vi "Serial_write_Read.vi"(8 "Error In":errorcluster caption="에러 입력", 10 "Command":string, 11 "VISA 리소스 이름":refnum<visa-resource-name>) -> (0 "Error Out":errorcluster caption="에러 출력", 2 "Response":T1, 3 "VISA 리소스 이름 출력":refnum<visa-resource-name>, 5 "bytes read":u32)   [LabVIEW 2015]
uses:
  MFC_Address.ctl
panel:
  out "연결된 문자열":string
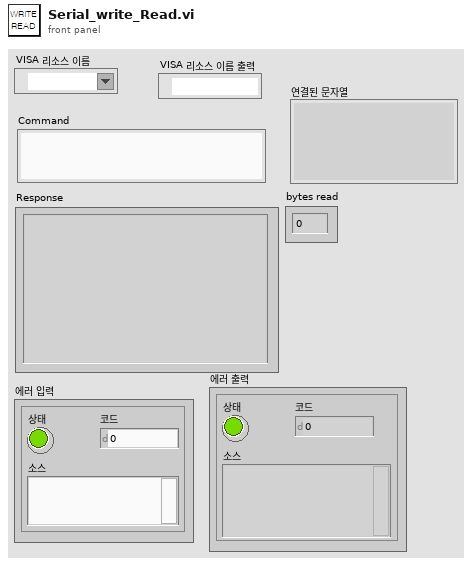
[diagram p1: front panel]
types:
  T1 = typedef "MFC_Address.ctl" = string
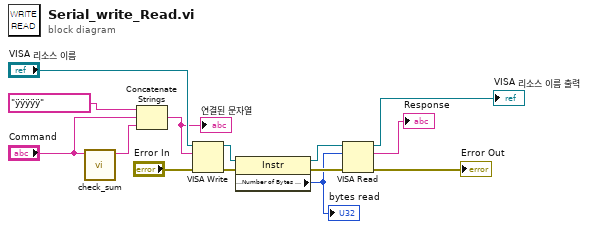
[diagram p0: block diagram]
diagram:
  n1 = call "check_sum.vi"("command"="Command") -> ("Check Sum"=w8:string)  [unwired: 10 in]
  n2 = Concatenate Strings("ÿÿÿÿÿ" ("문자열"), "Command", w8) -> (w6:string)
  "연결된 문자열" <- w6
  n3 = VISA Write(VISA resource name="VISA 리소스 이름", write buffer=w6, error in (no error)="Error In") -> (VISA resource name out=w11:refnum<visa-resource-name>, error out=w4:errorcluster)  [unwired: 1 out]
  n4 = property class="Instr"(reference=w11, error in=w4) -> (reference out=w14:refnum<visa-resource-name>, error out=w13:errorcluster, "Serial Settings:Number of Bytes at Serial Port"=w12:u32)
  "bytes read" <- w12
  n5 = VISA Read(VISA resource name=w14, byte count=w12, error in (no error)=w13) -> (VISA resource name out=→"VISA 리소스 이름 출력":refnum<visa-resource-name>, read buffer=→"Response":string, error out=→"Error Out":errorcluster)  [unwired: 1 out]
